vi "SAI_Query.vi"(0 "System no.":i32=1 min=1 max=4 step=1, 2 "Write to Global2?":bool, 3 "Invert order?":bool, 4 "SAI? ALL":bool, 5 "error in":errorcluster) -> (14 "Conn. axes":string[](array[string]), 19 "error out":errorcluster)   [LabVIEW 2020]
doc: "GCS 3.0\n=====\n\nSAI? (Get List of Current Axis Identifiers)\n\nDescription\nQueries the aliases (p. 94) for all axes of the controller.\n\nFormat\nSAI?[ ALL]\n\nArguments\nALL\nALL is only supported for compatibility reasons. The responses to SAI? without arguments and \nto SAI? ALL do not differ.\n\nResponse\n{<AxisID>LF}\n<AxisID>\nAn axis of the controller\nPossible values: Alias of the axis (p. 94) \n\nExample\n>>sai?\n<<AXIS_1\n<<AXIS_2\n>>sai? all\n<<AXIS_1\n<<AXIS_2\n\nNotes\nThe available axes are also contained in the response to USG? SYS (p. 80). \n\nUser command level\nUSR\n\n\nGCS 2.0\n=====\n\nReturns axis identifiers of all connected axes and writes them into Global2 (Array).vi. Required by Define connected axes.vi. If SAI? ALL is TRUE, all physically available axes are returned, no matter if configured or not. If SAI? ALL is TRUE, returned identifiers normally may not be written to Global2 (Array).vi. To write them to Global2 (Array).vi nevertheless, set \"Write to Global2?\" to TRUE. \n\nAnalog: Invert order should be FALSE, SAI? ALL must be FALSE\nC-702: Invert order should be TRUE, SAI? ALL must be FALSE\nC-848: Invert order should be TRUE, SAI? ALL must be FALSE\nC-880: Invert order should be TRUE, SAI? ALL must be FALSE to read all configured axis IDs and must be TRUE to get all physically defined axis IDs \nC-880K005: VI only supported when called through PI_Multix.vi, SAI? ALL must be FALSE\nE-516: Invert order should be FALSE, SAI? ALL must be FALSE\nE-816: Invert order should be FALSE, SAI? ALL must be FALSE\nAll other systems: Invert order should be FALSE, SAI? ALL is supported"
uses:
  Syntax.ctl
  Global1.vi
  Global2 (Array).vi
panel:
  # "SAI? (Get List of Current Axis Identifiers)\n\nQueries the aliases for all axes of the controller."
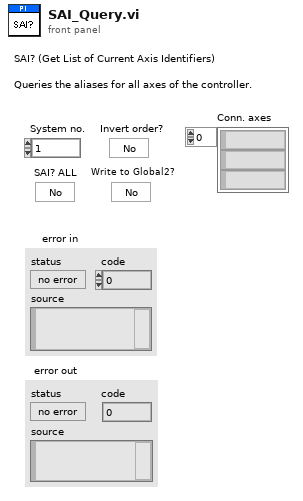
[diagram p1: front panel]
types:
  T1 = typedef "Syntax.ctl" = enum16{"GCS 1.0", "GCS 2.0", "GCS 3.0"}
  T2 = typedef "Controller names.ctl" = enum16{"None", "Analog", "C-702", "C-413", "C-414", "C-843", "C-843.PM", "C-844", "C-848", "C-865", "C-866", "C-867", "C-877", "C-880", "C-884", "C-885", "C-886", "C-887", "C-891", "E-135", "E-516", "E-517", "E-518", "E-709", "E-710", "E-712", "E-725", "E-727", "E-753", "E-754", "E-755", "E-761", "E-816", "E-861", "E-870", "E-871", "E-872", "E-873", "E-874", "F-206", "HydraPollux", "M-840", "M-850", "M-8X0", "Mercury", "Mercury_GCS", "PI_GCS2"}
  T3 = cluster{"Conn. axes":string[], "Controller name":T2}[]
  T4 = cluster{"Conn. axes":string[], "Controller name":T2}
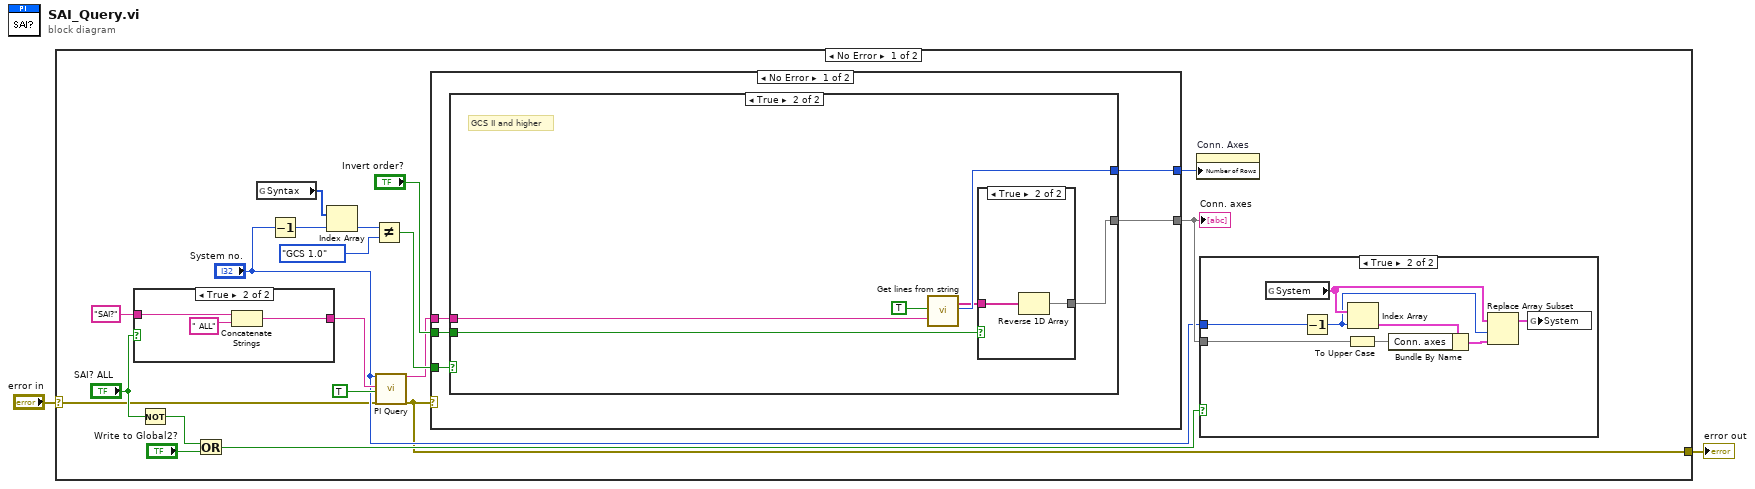
[diagram p0: block diagram]
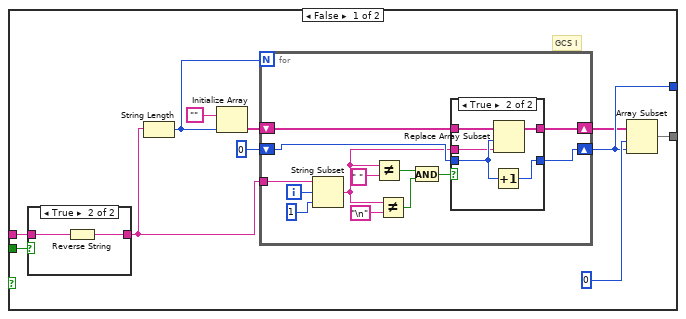
[diagram p3: hidden frame]
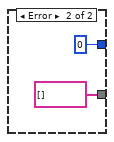
[diagram p7: hidden frame]
diagram:
  n1 = case shown="No Error" "error in" {
    selector: "error in" -> [w6 w84]
    tunnel: [w4 w84] -> w2
    frame No Error {
      n2 = case shown="True" "SAI? ALL" {
        tunnel: "SAI?" -> [w80 w82]
        tunnel: [w80 w81] -> w17
        frame False {
        }
        frame True {
          n3 = Concatenate Strings(w82, " ALL") -> (w81:string)
        }
      }
      n4 = Not(x="SAI? ALL") -> (.not. x?=w8:bool)
      n5 = Or(x=w8, y="Write to Global2?") -> (x .or. y?=w7:bool)
      n6 = global read "Global1.vi" "Syntax"() -> (w13:T1[])
      n7 = Decrement(x="System no.") -> (x-1=w14:i32)
      n8 = Index Array(array=w13, index=w14) -> (element=w15:T1)
      n9 = Not Equal?(x=w15, y=Syntax."GCS 1.0") -> (x != y?=w11:bool)
      n10 = call "PI Query.vi"("System no."="System no.", "String to send"=w17, "Attach termination char.?"=TRUE ("Attach Linefeed?"), "error in"=w6) -> ("String read"=w5:string, "error out"=w4:errorcluster)  [unwired: 3 in, 11 out]
      n11 = case shown="No Error" w4 {
        tunnel: "Invert order?" -> [w31 _]
        tunnel: w5 -> [w32 _]
        tunnel: [w34 0 ("Array size out")] -> w19
        tunnel: [w33 string[] [] ("Strings")] -> w16
        tunnel: w11 -> [w30 _]
        frame No Error {
          n12 = case shown="True" w30 {
            tunnel: [w40 w71] -> w34
            tunnel: [w38 w69] -> w33
            tunnel: w32 -> [w37 w73]
            tunnel: w31 -> [w35 w72]
            frame False {
              # "GCS I"
              n13 = case shown="True" w35 {
                tunnel: w37 -> [w46 w48]
                tunnel: [w46 w47] -> w36
                frame False {
                }
                frame True {
                  n14 = Reverse String(1:w48) -> (0:w47:string)
                }
              }
              n15 = String Length(string=w36) -> (length=w44:i32)
              n16 = Initialize Array("" ("Element Data"), w44) -> (w42:string[])
              n17 = for {
                N: w44 -> [_]
                tunnel: w36 -> [w61]
                shift-right: [w54] -> w39
                shift-left: w42 -> [w55]
                shift-right: [w57] -> w40
                shift-left: 0 -> [w56]
                i -> [w59]
                n18 = String Subset(string=w61, offset (0)=w59, length (rest)=1 ("length")) -> (substring=w53:string)
                n19 = Not Equal?(x=w53, y=" ") -> (x != y?=w51:bool)
                n20 = Not Equal?(x=w53, y="\n") -> (x != y?=w50:bool)
                n21 = And(x=w51, y=w50) -> (x .and. y?=w49:bool)
                n22 = case shown="True" w49 {
                  tunnel: [w63 w68] -> w57
                  tunnel: w56 -> [w63 w66]
                  tunnel: w55 -> [w62 w67]
                  tunnel: w53 -> [_ w65]
                  tunnel: [w62 w64] -> w54
                  frame False {
                  }
                  frame True {
                    n23 = Increment(x=w66) -> (x+1=w68:i32)
                    n24 = Replace Array Subset(array=w67, new element=w65, index=w66) -> (w64:string[])
                  }
                }
              }
              n25 = Array Subset(array=w39, index=0 ("Array Index"), length=w40) -> (w38:string[])
            }
            frame True {
              # "GCS II and higher"
              n26 = call "Get lines from string.vi"("Cut spaces?"=TRUE, "Input string"=w73) -> ("Strings"=w70:string[], "Array size out"=w71:i32)  [unwired: 1 in, 15 out]
              n27 = case shown="True" w72 {
                tunnel: w70 -> [w75 w77]
                tunnel: [w75 w76] -> w69
                frame False {
                }
                frame True {
                  n28 = Reverse 1D Array(array=w77) -> (reversed array=w76:string[])
                }
              }
            }
          }
        }
        frame Error {
        }
      }
      "Conn. axes" <- w16
      n29 = property on="Conn. Axes" class="Arr (strict)"("Number of Rows"=w19) -> ()  [unwired: 2 in, 2 out]
      n30 = case shown="True" w7 {
        tunnel: w16 -> [_ w25]
        tunnel: "System no." -> [_ w23]
        frame False {
        }
        frame True {
          n31 = global read "Global2 (Array).vi" "System"() -> (w28:T3)
          n32 = Decrement(x=w23) -> (x-1=w27:i32)
          n33 = To Upper Case(1:w25) -> (0:w22:string[])
          n34 = Index Array(array=w28, index=w27) -> (element=w26:T4)
          n35 = Bundle By Name(cluster=w26, "Conn. axes"=w22) -> (w24:T4)
          n36 = Replace Array Subset(array=w28, new element=w24, index=w27) -> (w29:T3)
          n37 = global write "Global2 (Array).vi" "System"(w29) -> ()
        }
      }
    }
    frame Error {
    }
  }
  "error out" <- w2
